vi "Write Bits.vi"(8 "error in (no error)":errorcluster, 9 "Bits Data":bool[](array[boolean]), 10 "Address":u16=65535 format="%.0x", 11 "Port Selection Info":T1={"Port Name"="", "Amplifier Num"=1, "Baud Rate"=38400, "Char Formation"=enum."0"} {"Baud Rate" items=["38400"=38400, "19200"=19200, "9600"=9600, "115200"=0]; "Amplifier Num" max=31}) -> (0 "error out":errorcluster, 3 "Port Selection Info Out":T1={"Port Name"="", "Amplifier Num"=1, "Baud Rate"=38400, "Char Formation"=enum."0"} {"Baud Rate" items=["38400"=38400, "19200"=19200, "9600"=9600, "115200"=0]; "Amplifier Num" max=31})   [LabVIEW 2014, in "ALPHA5 RS485.lvlib"]
uses:
  ALPHA5 RS485.lvlib
  typedefs/Port Selection Info.ctl
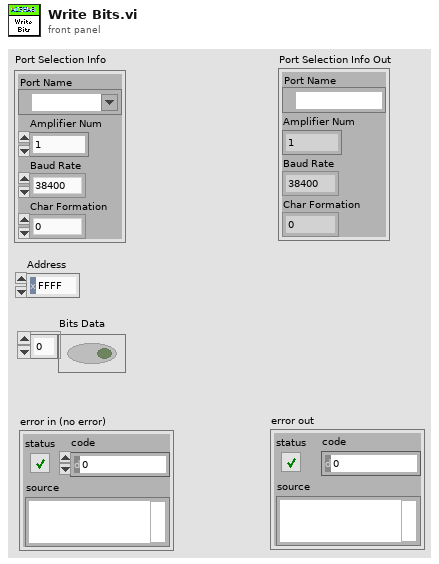
[diagram p1: front panel]
types:
  T1 = typedef "ALPHA5 RS485.lvlib/Port Selection Info.ctl" = cluster{"Port Name":refnum<visa-resource-name>, "Amplifier Num":u8, "Baud Rate":u32, "Char Formation":enum16{"0", "1", "2", "3", "4", "5"}}
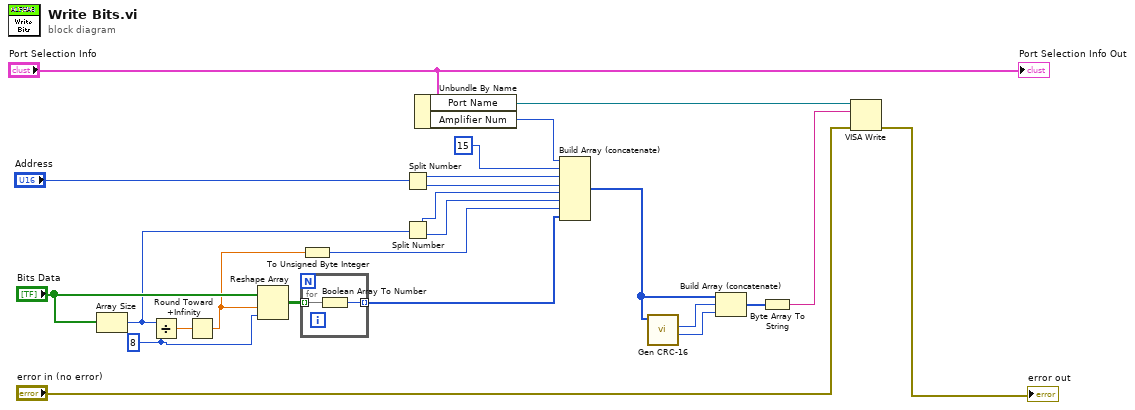
[diagram p0: block diagram]
diagram:
  w6 = 8 ("y")
  n1 = Array Size(array="Bits Data") -> (size(s)=w5:i32)
  n2 = Divide(x=w5, y=w6) -> (x/y=w8:dbl)
  n3 = Round Toward +Infinity(x=w8) -> (ceil(x): smallest int >= x=w3:dbl)
  n4 = Reshape Array("Bits Data", w3, w6) -> (w4:bool[][])
  n5 = for {
    tunnel: w4 -> [w26] mode=indexing
    tunnel: [w25] -> w1 mode=indexing
    n6 = Boolean Array To Number(Boolean array=w26) -> (number=w25:u32)
  }
  n7 = To Unsigned Byte Integer(number=w3) -> (unsigned 8bit integer=w2:u8)
  n8 = Split Number(x="Address") -> (hi(x)=w18:u8, lo(x)=w17:u8)
  n9 = Split Number(x=w5) -> (hi(x)=w16:u16, lo(x)=w15:u16)
  n10 = Unbundle By Name("Port Selection Info") -> ("Port Name"=w10:refnum<visa-resource-name>, "Amplifier Num"=w19:u8)
  n11 = Build Array (concatenate)(w19, u8 15 ("FC"), w18, w17, w16, w15, w2, w1) -> (w11:u32[])
  n12 = call "Gen CRC-16.vi"("Data In"=w11) -> ("CRC-16-H"=w13:u8, "CRC-16-L"=w14:u8)  [unwired: 7 in, 2 out]
  n13 = Build Array (concatenate)(w11, w14, w13) -> (w12:u32[])
  n14 = Byte Array To String(unsigned byte array=w12) -> (string=w9:string)
  n15 = VISA Write(VISA resource name=w10, write buffer=w9, error in (no error)="error in (no error)") -> (error out=→"error out":errorcluster)  [unwired: 2 out]
  "Port Selection Info Out" <- "Port Selection Info"
